vi "replace_or_add_element_to_ItemNames.vi"(6 "element":string, 9 "column":i32, 10 "row":i32, 11 "ItemNames_in":string[][](array[string])) -> (3 "ItemNames_out":string[][](array[string]))   [LabVIEW 2019]
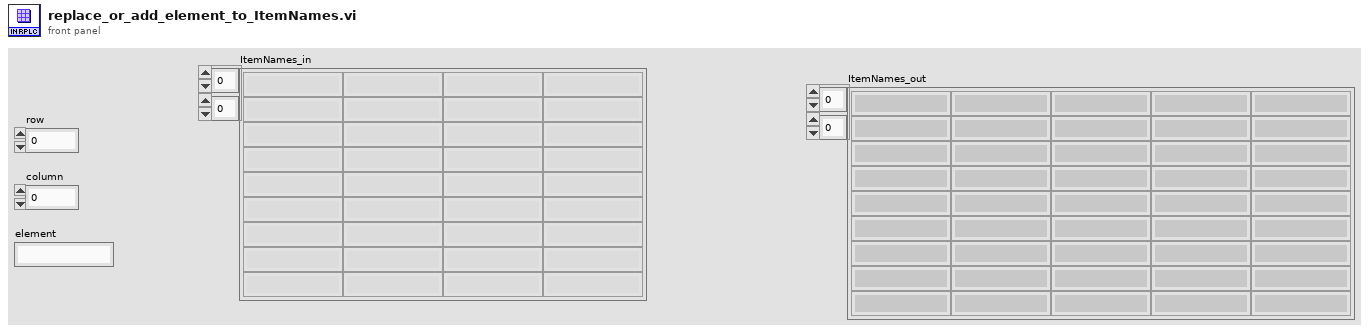
[diagram p1: front panel]
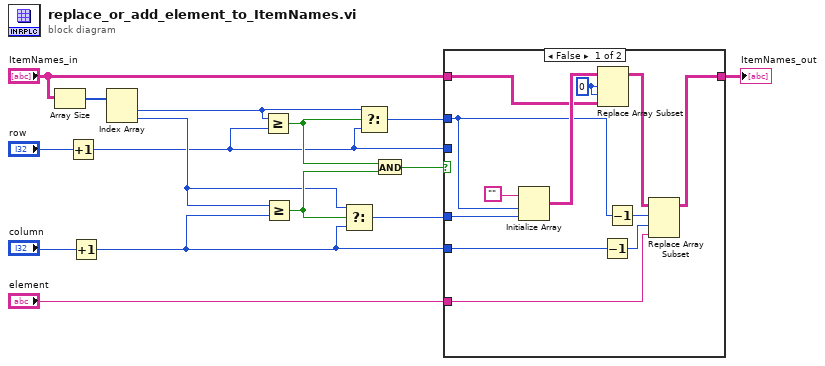
[diagram p0: block diagram]
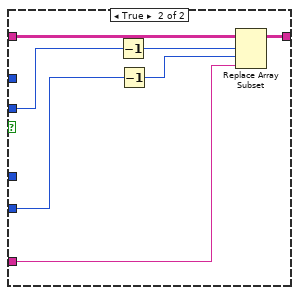
[diagram p2: hidden frame]
diagram:
  n1 = Array Size(array="ItemNames_in") -> (size(s)=w12:i32[])
  n2 = Increment(x="row") -> (x+1=w4:i32)
  n3 = Increment(x="column") -> (x+1=w1:i32)
  n4 = Index Array(array=w12) -> (element #1=w9:i32, element #2=w6:i32)  [unwired: 2 in]
  n5 = Greater Or Equal?(x=w9, y=w4) -> (x >= y?=w10:bool)
  n6 = Greater Or Equal?(x=w6, y=w1) -> (x >= y?=w7:bool)
  n7 = Select(t=w6, s=w7, f=w1) -> (s? t:f=w5:i32)
  n8 = Select(t=w9, s=w10, f=w4) -> (s? t:f=w8:i32)
  n9 = And(x=w10, y=w7) -> (x .and. y?=w11:bool)
  n10 = case shown="False" w11 {
    tunnel: "element" -> [w22 w34]
    tunnel: [w23 w33] -> w14
    tunnel: "ItemNames_in" -> [w20 w32]
    tunnel: w8 -> [w16 _]
    tunnel: w5 -> [w26 _]
    tunnel: w4 -> [_ w30]
    tunnel: w1 -> [w17 w29]
    frame False {
      w25 = 0 ("index (row)")
      n11 = Initialize Array("", w16, w26) -> (w21:string[][])
      n12 = Replace Array Subset(array=w21, new element=w20, index (row)=w25, index (col)=w25) -> (w24:string[][])
      n13 = Decrement(x=w17) -> (x-1=w18:i32)
      n14 = Decrement(x=w16) -> (x-1=w19:i32)
      n15 = Replace Array Subset(array=w24, new element=w22, index (row)=w19, index (col)=w18) -> (w23:string[][])
    }
    frame True {
      n16 = Decrement(x=w30) -> (x-1=w31:i32)
      n17 = Decrement(x=w29) -> (x-1=w28:i32)
      n18 = Replace Array Subset(array=w32, new element=w34, index (row)=w31, index (col)=w28) -> (w33:string[][])
    }
  }
  "ItemNames_out" <- w14
